vi "Phase Shift Caluclate.vi"(6 "Board mode":enum16{"M*1", "M*N"}(ring), 9 "Pitch angle(phi)":dbl, 11 "Azimuth angle(theta)":dbl) -> (3 "phase shift":dbl)   [LabVIEW 2014]
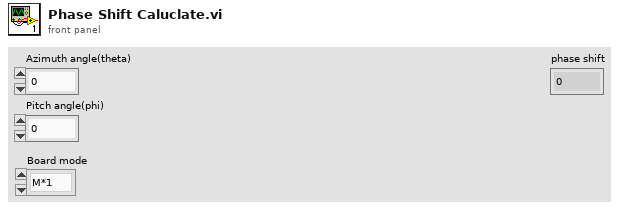
[diagram p1: front panel]
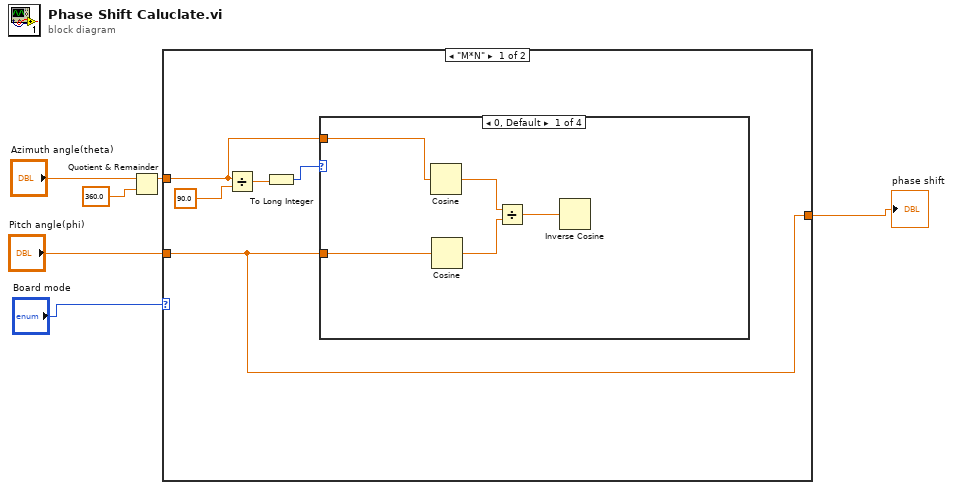
[diagram p0: block diagram]
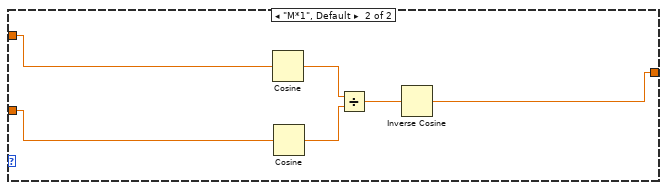
[diagram p5: hidden frame]
diagram:
  n1 = Quotient & Remainder(x="Azimuth angle(theta)", y=360.0) -> (x-y*floor(x/y)=w4:dbl)  [unwired: 1 out]
  n2 = case shown="\"M*N\"" "Board mode" {
    tunnel: w4 -> [w8 w19]
    tunnel: "Pitch angle(phi)" -> [w7 w18]
    tunnel: [w7 w17] -> w2
    frame "M*N" {
      n3 = Divide(x=w8, y=90.0) -> (x/y=w10:dbl)
      n4 = To Long Integer(number=w10) -> (32bit integer=w9:i32)
      n5 = case shown="0, Default" w9 {
        tunnel: w8 -> [w13 _ _ _]
        tunnel: w7 -> [w12 _ _ _]
        frame 0, Default {
          n6 = Cosine(x=w13) -> (cos(x)=w14:dbl)
          n7 = Cosine(x=w12) -> (cos(x)=w15:dbl)
          n8 = Divide(x=w14, y=w15) -> (x/y=w16:dbl)
          n9 = Inverse Cosine(1:w16) -> ()  [unwired: 1 out]
        }
        frame 1 {
        }
        frame 2 {
        }
        frame 3, 4 {
        }
      }
    }
    frame "M*1", Default {
      n10 = Cosine(x=w19) -> (cos(x)=w22:dbl)
      n11 = Cosine(x=w18) -> (cos(x)=w21:dbl)
      n12 = Divide(x=w22, y=w21) -> (x/y=w20:dbl)
      n13 = Inverse Cosine(1:w20) -> (0:w17:dbl)
    }
  }
  "phase shift" <- w2
